vi "Cikautxo Intermix if VI is running stop VI.vi"(8 "error in (no error)":errorcluster, 11 "VI in":refnum<vi>) -> (0 "error out":errorcluster, 3 "VI out":refnum<vi>)   [LabVIEW 2017]
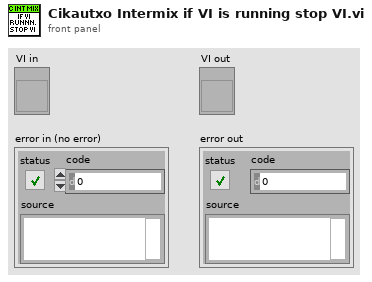
[diagram p1: front panel]
types:
  T1 = enum32{"Bad", "Idle", "Run top level", "Running"}
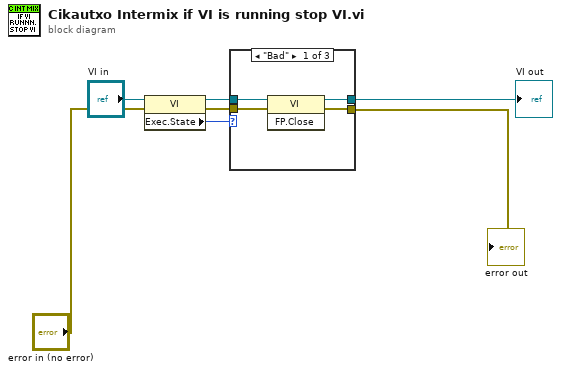
[diagram p0: block diagram]
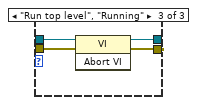
[diagram p3: hidden frame]
diagram:
  n1 = property class="VI"(reference="VI in", error in="error in (no error)") -> (reference out=w5:refnum<vi>, error out=w4:errorcluster, "Exec.State"=w3:T1)
  n2 = case shown="\"Bad\"" w3 {
    tunnel: w4 -> [w9 w12 w17]
    tunnel: w5 -> [w11 w13 w16]
    tunnel: [w10 w13 w15] -> w6
    tunnel: [w8 w12 w14] -> w7
    frame "Bad" {
      n3 = invoke class="VI" method="FP.Close"(reference=w11, error in=w9) -> (reference out=w10:refnum<vi>, error out=w8:errorcluster)  [unwired: 1 in, 1 out]
    }
    frame "Idle", Default {
    }
    frame "Run top level", "Running" {
      n4 = invoke class="VI" method="Abort VI"(reference=w16, error in=w17) -> (reference out=w15:refnum<vi>, error out=w14:errorcluster)  [unwired: 1 in, 1 out]
    }
  }
  "error out" <- w7
  "VI out" <- w6
